vi "Master Config to String.vi"(10 "Filter Sequences":T1[](array[typedef]), 11 "Gas Mixtures":T2[](array[typedef]) {"ADC Gains" items=["0"=0, "3"=3, "4"=4, "5"=5, "6"=6, "7"=7]}) -> (2 "Filter":string[][](array[string]), 3 "Gas":string[][](array[string]))   [LabVIEW 2015]
uses:
  Tests/Controls/Gas Mixture.ctl
  CAN Communication/PAS/Typedefs/ADC Gains.ctl
  Tests/Controls/Filter Sequence.ctl
  CAN Communication/PAS/PAS.lvclass
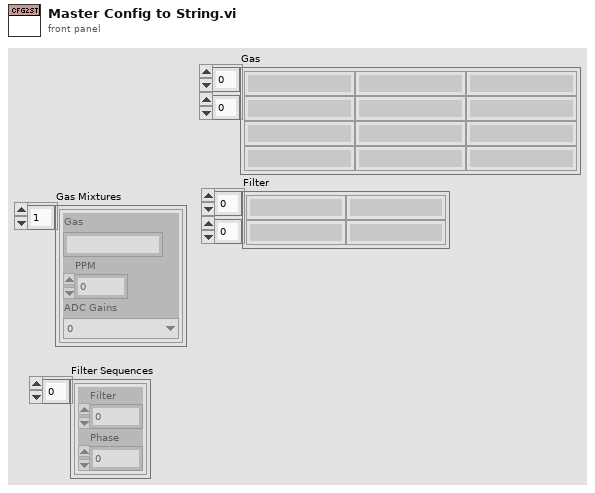
[diagram p1: front panel]
types:
  T1 = typedef "Filter Sequence.ctl" = cluster{"Filter":u8, "Phase":dbl}
  T2 = typedef "Gas Mixture.ctl" = cluster{"Gas":string, "PPM":dbl, "ADC Gains":T3}
  T3 = typedef "PAS.lvclass/ADC Gains.ctl" = u16
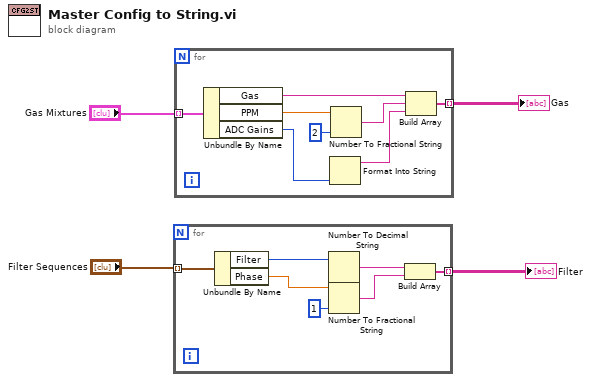
[diagram p0: block diagram]
diagram:
  n1 = for {
    tunnel: "Filter Sequences" -> [w11] mode=indexing
    tunnel: [w9] -> w1 mode=indexing
    n2 = Unbundle By Name(w11) -> ("Filter"=w7:u8, "Phase"=w10:dbl)
    n3 = Number To Decimal String(number=w7) -> (decimal integer string=w6:string)  [unwired: 1 in]
    n4 = Number To Fractional String(number=w10, precision (6)=i16 1) -> (F-format string=w5:string)  [unwired: 2 in]
    n5 = Build Array(w6, w5) -> (w9:string[])
  }
  "Filter" <- w1
  n6 = for {
    tunnel: "Gas Mixtures" -> [w19] mode=indexing
    tunnel: [w12] -> w3 mode=indexing
    n7 = Unbundle By Name(w19) -> ("Gas"=w18:string, "PPM"=w17:dbl, "ADC Gains"=w15:T3)
    n8 = Format Into String(w15) -> (resulting string=w13:string)  [unwired: 3 in, 1 out]
    n9 = Number To Fractional String(number=w17, precision (6)=i16 2) -> (F-format string=w14:string)  [unwired: 2 in]
    n10 = Build Array(w18, w14, w13) -> (w12:string[])
  }
  "Gas" <- w3
